vi "Joystick - Array to Cluster.vi"(1 "Axes":dbl[](array[numeric])) -> (0 "Axes [Cluster]":T1)   [LabVIEW 2015]
uses:
  Logitech Attack 3 Axis Map.ctl
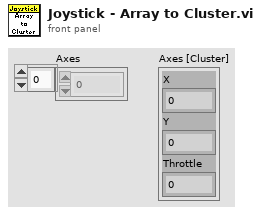
[diagram p1: front panel]
types:
  T1 = typedef "Logitech Attack 3 Axis Map.ctl" = cluster{"X":dbl, "Y":dbl, "Throttle":dbl}
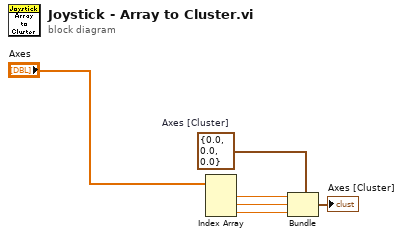
[diagram p0: block diagram]
diagram:
  w2 = T1 {"X"=0.0, "Y"=0.0, "Throttle"=0.0}  # Axes [Cluster]
  n1 = Index Array(array="Axes") -> (element #1=w3:dbl, element #2=w4:dbl, element #3=w5:dbl)  [unwired: 3 in]
  n2 = Bundle(cluster=w2, "X"=w3, "Y"=w4, "Throttle"=w5) -> (→"Axes [Cluster]":T1)
